vi "IEPE - Continuous  Input_tet.vi"() -> ()   [LabVIEW 2025]
doc: "This example demonstrates how to continuously acquire buffered acceleration, sound pressure, or force measurements from IEPE sensors using a DAQmx device.\n\nFor instructions on how to connect your signals to the DAQ device, refer to your device documentation."
uses:
  <vilib>/Math Plots/3D Math Plots/3D Contour/3D Contour XCtrl/3D Contour.xctl
  <vilib>/Utility/error.llb/DialogType.ctl
  <vilib>/DAQmx/read.llb/DAQmx Read (Analog 1D Wfm NChan NSamp).vi
  <vilib>/DAQmx/miscellaneous.llb/DAQmx Fill In Error Info.vi
  <vilib>/DAQmx/configure/trigger.llb/DAQmx Start Trigger (Digital Edge).vi
  <vilib>/DAQmx/configure/timing.llb/DAQmx Timing (Sample Clock).vi
  <vilib>/DAQmx/configure/task.llb/DAQmx Configure Logging (TDMS).vi
  <vilib>/DAQmx/create/channels.llb/DAQmx Create Channel (AI-Sound Pressure-Microphone).vi
  <vilib>/DAQmx/create/channels.llb/DAQmx Create Channel (AI-Force-IEPE Sensor).vi
  <vilib>/DAQmx/create/channels.llb/DAQmx Create Channel (AI-Acceleration-Accelerometer).vi
  <vilib>/DAQmx/configure/trigger.llb/DAQmx Start Trigger (Analog Edge).vi
  <vilib>/DAQmx/configure/trigger.llb/DAQmx Start Trigger (Time).vi
  <vilib>/Math Plots/3D Math Plots/3D Contour/3D Contour Datatype/Public/Plot Helper (Vector).vi
  <vilib>/Waveform/WDTOps.llb/WDT Waveform Duration DBL.vi
  <vilib>/Waveform/WDTOps.llb/WDT Append Waveforms DBL.vi
  <resource>/objmgr/daqmx.rc
  <vilib>/Math Plots/3D Math Plots/3D Contour/3D Contour Datatype/3D Contour Datatype.lvclass
panel:
  in  "last order plot":sgl
  in  "rotation speed":sgl
  out "3D-Kontur":refnum<class "3D Plot Datatype.lvclass">[](xcontrol)
  in  "filename":string
  in  "Dateipfad":path
  in  "on hold time (s)":u32=900
  out "FFT":cluster{dbl, "freq_step":dbl, "abs_FFT":dbl[]}(graph)
  in  "duration (s) control":dbl=30.0
  out "current duration":dbl caption="Dauer" format="%0.2f"
  in  "Trigger Type":T1(tab)
  in  "Digital Start Trigger Edge":i32(ring)=10280 caption="Edge" items=["Rising"=10280, "Falling"=10171]
  in  "Digital Start Trigger Source":tag="/Dev1/PFI0" caption="Source"
  in  "Digital Pause Trigger Pause When":i32(ring)=10192 caption="Pause When" items=["High"=10192, "Low"=10214]
  in  "Digital Pause Trigger Source":tag="/Dev1/PFI0" caption="Source"
  in  "Analog Start Trigger Level":dbl caption="Level" format="%0.2f"
  in  "Analog Start Trigger Hysteresis":dbl caption="Hysteresis" format="%.2f"
  in  "Analog Start Trigger Slope":i32(ring)=10280 caption="Slope" items=["Rising"=10280, "Falling"=10171]
  in  "Analog Start Trigger Source":string="APFI0" caption="Source"
  in  "Analog Pause Trigger Source":string="APFI0" caption="Source"
  in  "Analog Pause Trigger Pause When":i32(ring)=10093 caption="Pause When" items=["Above Level"=10093, "Below Level"=10107]
  in  "Analog Pause Trigger Level":dbl caption="Level" format="%.2f"
  in  "When":timestamp
  in  "Select Time\nManually":bool
  in  "IEPE Current Value (A)":dbl=0.004
  in  "IEPE Excitation Source":i32(ring)=10200 items=["Internal"=10200, "External"=10167, "None"=10230]
  in  "Terminal Configuration":i32(ring)=-1 items=["default"=-1, "RSE"=10083, "NRSE"=10078, "Differential"=10106, "Pseudodifferential"=12529]
  in  "Physical Channel":tag="cDAQ3Mod2/ai0"
  in  "Task Type":T2(tab)
  in  "Min Acceleration":dbl=-100.0
  in  "Max Acceleration":dbl=100.0
  in  "Sensitivity":dbl=50.0
  in  "Acceleration Units":i32(ring)=10186 items=["g"=10186, "m/s^2"=12470, "in/s^2"=12471, "From Custom Scale"=10065]
  in  "Sensitivity Units":i32(ring)=12509 items=["mVolts/g"=12509, "Volts/g"=12510]
  in  "Max Sound Pressure Level (dB)":dbl=120.0
  in  "Sound Pressure Units":i32(ring)=10081 items=["Pascals"=10081, "From Custom Scale"=10065]
  in  "Microphone Sensitivity":dbl=10.0
  in  "Sensitivity":dbl=50.0
  in  "Min Force":dbl=-100.0
  in  "Max Force":dbl=100.0
  in  "Sensitivity Units":i32(ring)=15891 items=["mVolts/N"=15891, "mVolts/lb"=15892]
  in  "Force Units":i32(ring)=15875 items=["Newtons"=15875, "Pounds"=15876, "From Custom Scale"=10065]
  in  "Stop":bool
  out "Waveform Graph":waveform(dbl)[](graph)
  in  "TDMS File Path":path
  in  "Samples per Loop":i32=100
  in  "Sample Rate":dbl=1000.0
  in  "Sample Clock Source":tag="OnboardClock"
  out "Actual Sample Rate":dbl=1000.0000111176631 format="%0.2f"
  in  "Logging Mode":i32(ring)=10231 items=["Off"=10231, "Log and Read"=15842]
  # "Channel Settings"
  # "Acquired Data"
  # "Trigger Settings"
  # "Timing Settings"
  # "Logging Settings"
  # "To enable triggers, select a tab above, and configure the settings.\n\nNot all hardware supports all trigger types. Refer to your device documentation for more information."
  # "This trigger type is not supported in continuous sample timing. \n\nRefer to your device documentation for more information on which triggers are supported."
  # "This trigger type is not supported in continuous sample timing. \n\nRefer to your device documentation for more information on which triggers are supported."
  # "If time is not manually set, task will begin after 10 seconds"
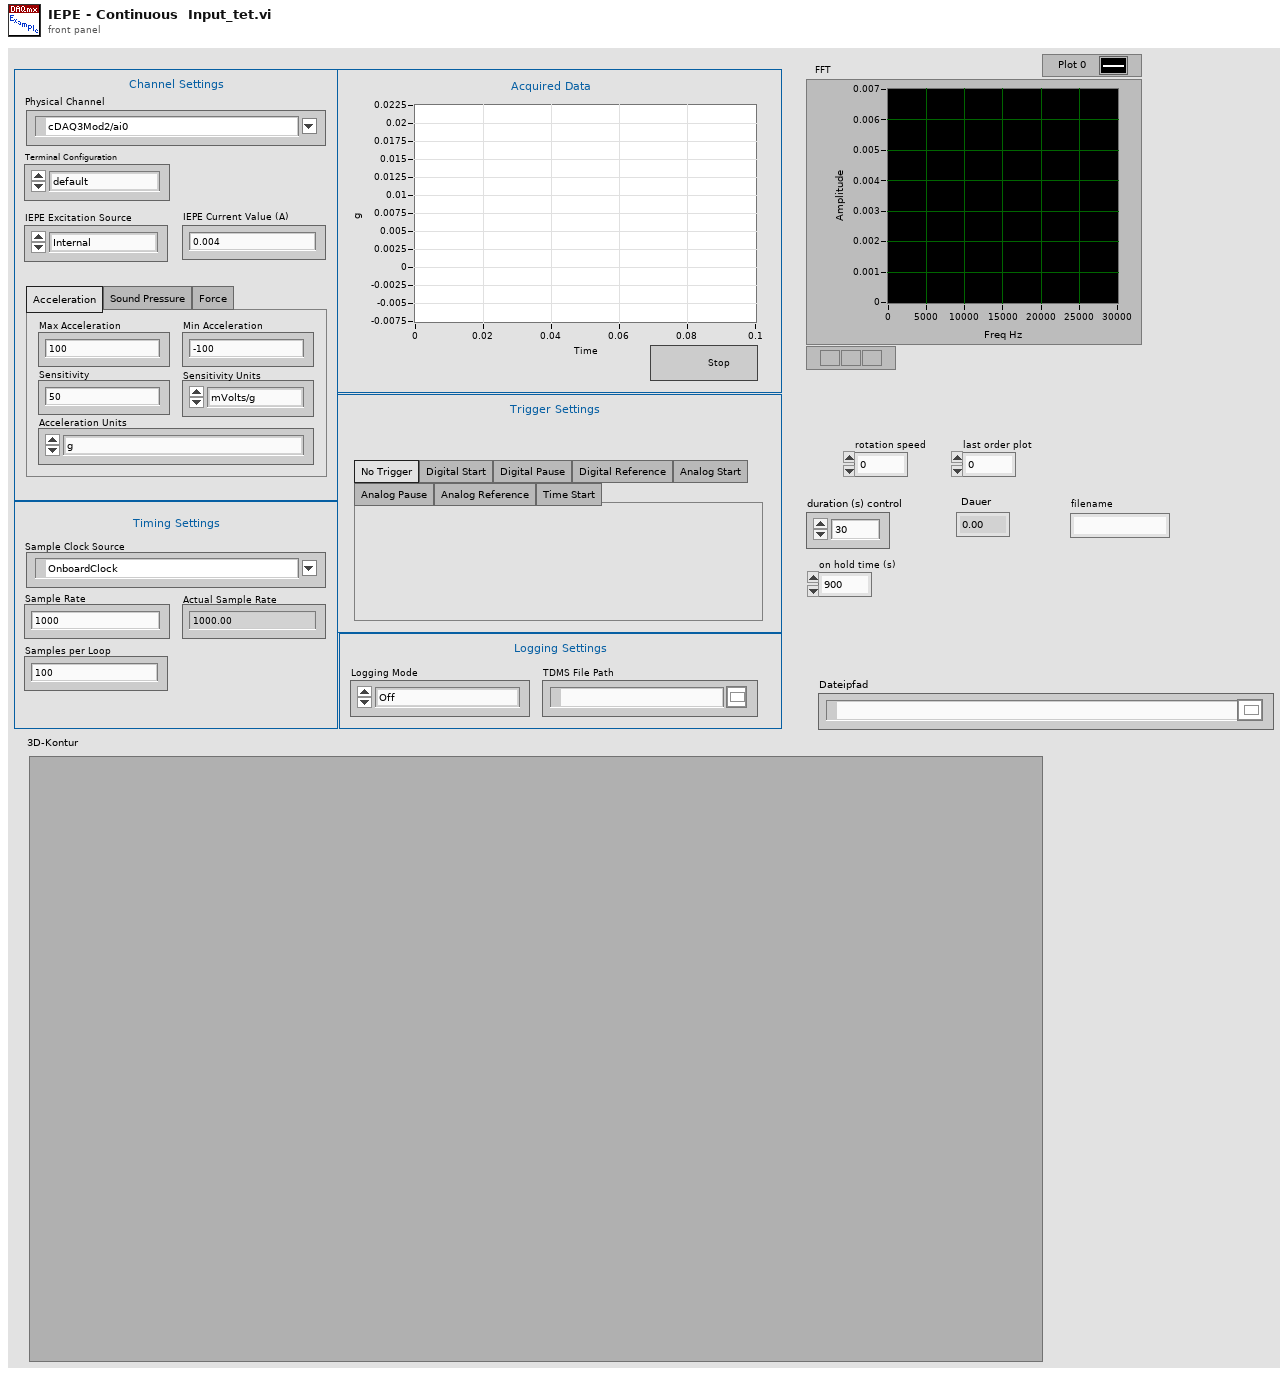
[diagram p1: front panel]
types:
  T1 = enum32{"No Trigger", "Digital Start", "Digital Pause", "Digital Reference", "Analog Start", "Analog Pause", "Analog Reference", "Time Start"}
  T2 = enum32{"Acceleration", "Sound Pressure", "Force"}
  T3 = typedef "DialogType.ctl" = u16
  T4 = cluster{"abs_FFT":dbl[], "frequencies":dbl[], "Huell_spec":dbl[], "Envelope":dbl[], "freq_step":dbl, "duration":dbl}
  T5 = enum16{"open", "open or create", "create or replace", "create", "open (read-only)"}
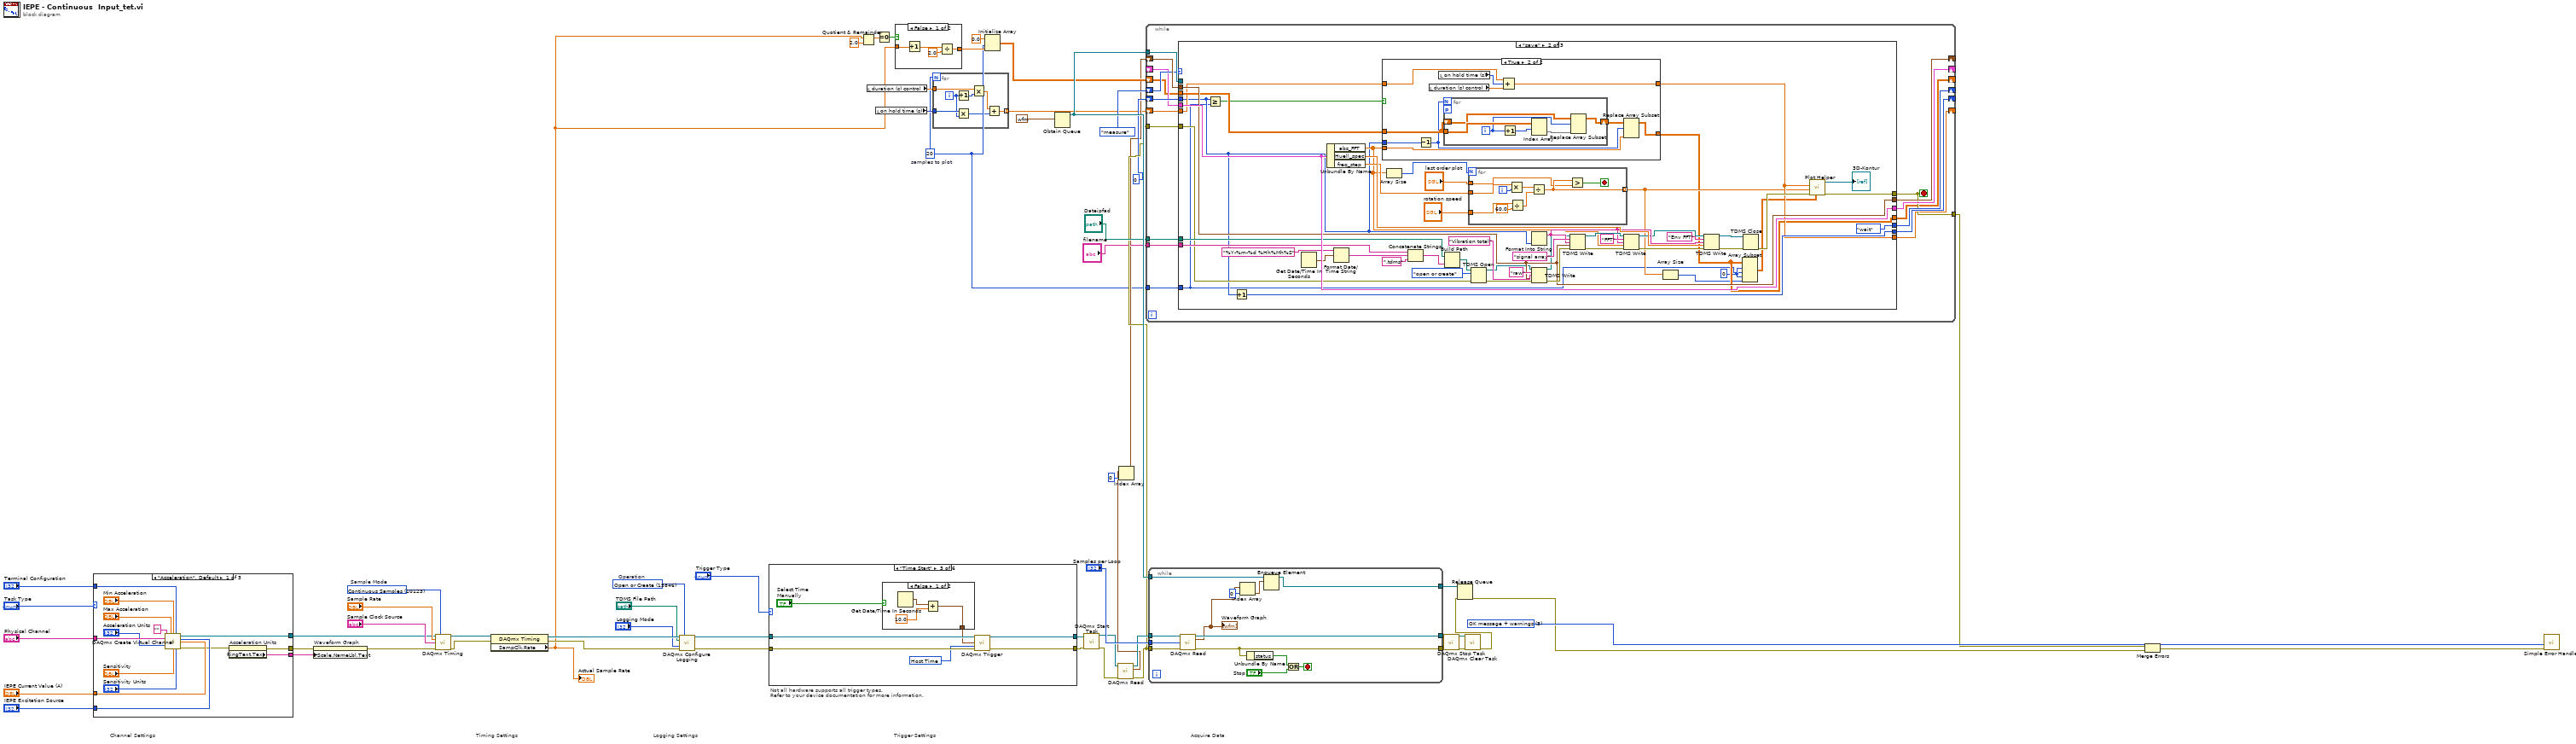
[diagram p0: block diagram]
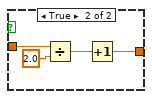
[diagram p2: hidden frame]
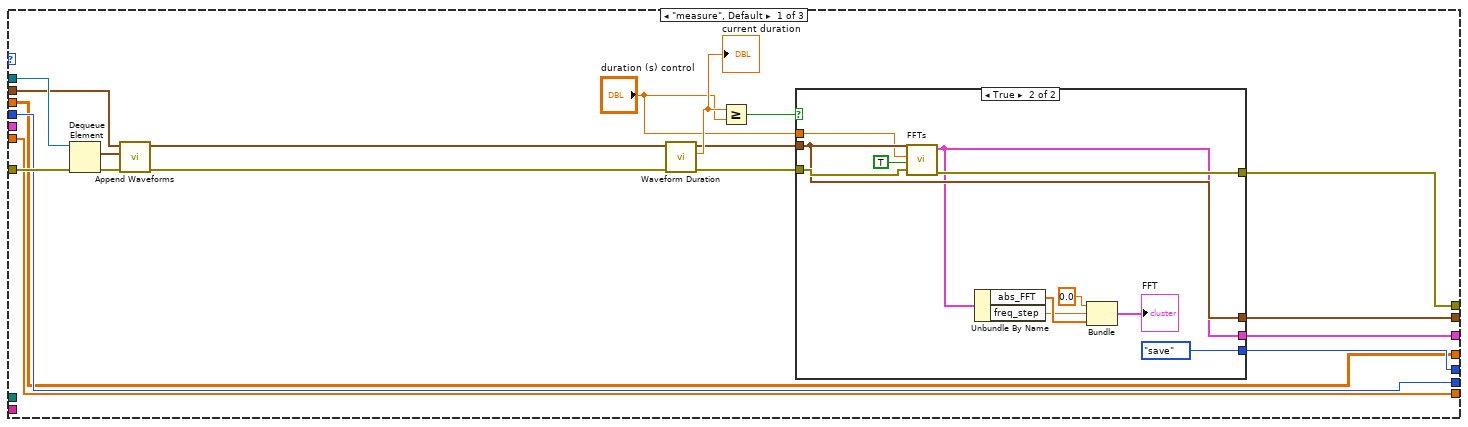
[diagram p3: hidden frame]
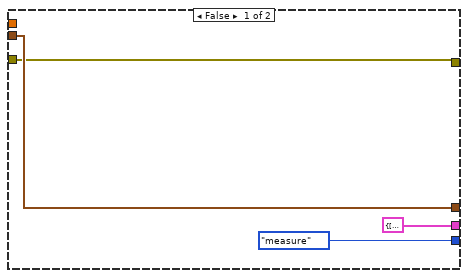
[diagram p4: hidden frame]
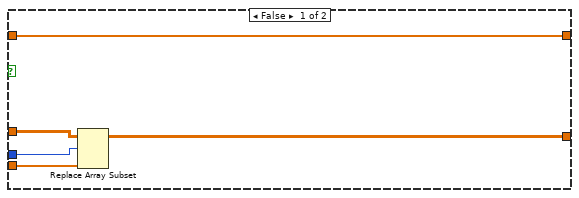
[diagram p5: hidden frame]
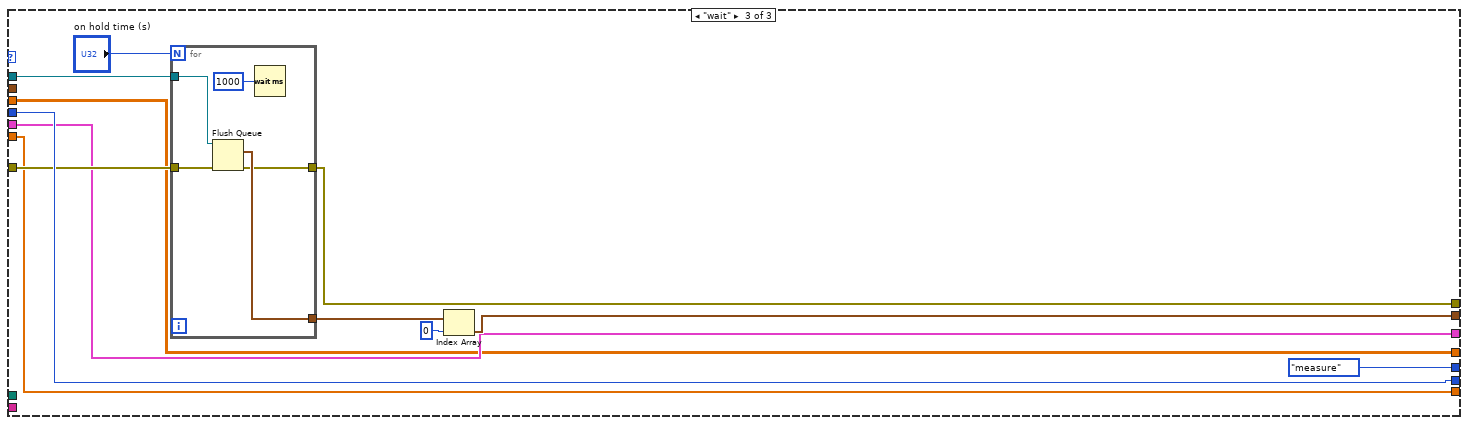
[diagram p6: hidden frame]
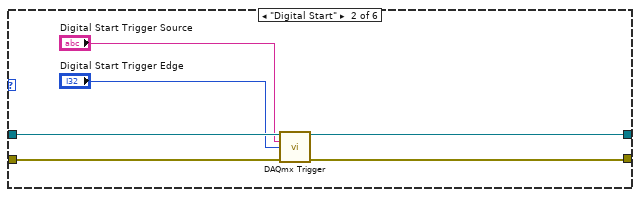
[diagram p8: hidden frame]
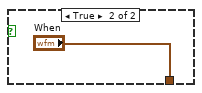
[diagram p9: hidden frame]
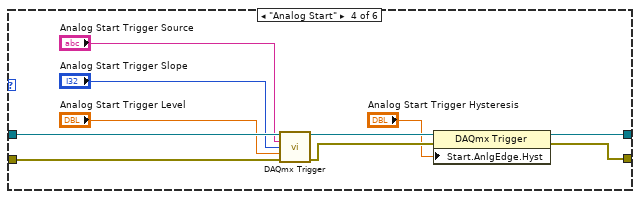
[diagram p10: hidden frame]
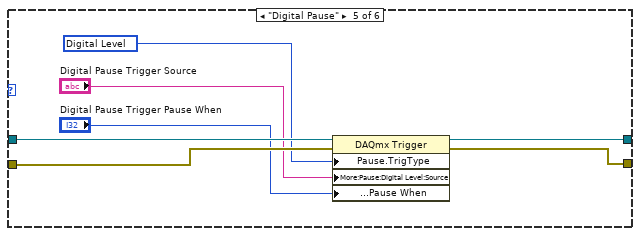
[diagram p11: hidden frame]
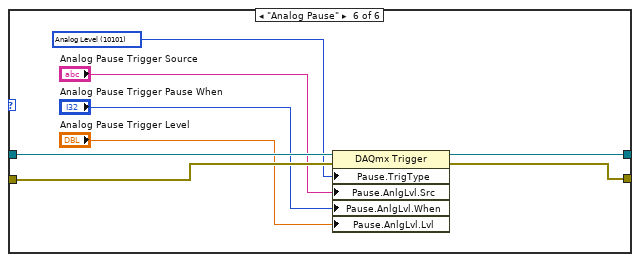
[diagram p12: hidden frame]
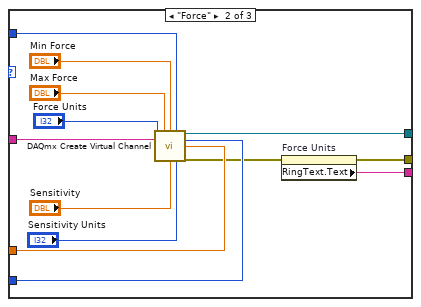
[diagram p13: hidden frame]
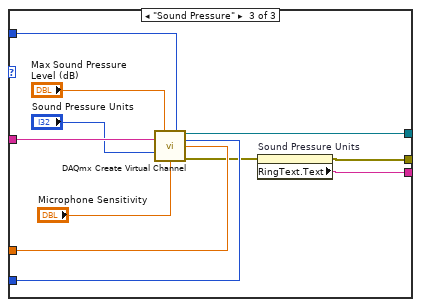
[diagram p14: hidden frame]
diagram:
  w1 = 20  # samples to plot
  w36 = T3 3 items=["no dialog", "OK message", "continue or stop message", "OK message + warnings", "continue/stop + warnings"] ("type of dialog (OK msg:1)")
  w54 = 15846 items=["Open"=10437, "Open or Create"=15846, "Create or Replace"=15847, "Create"=15848]  # Operation
  w57 = 10123 items=["Finite Samples"=10178, "Continuous Samples"=10123, "Hardware Timed Single Point"=12522]  # Sample Mode
  # "Trigger Settings"
  # "Not all hardware supports all trigger types.\nRefer to your device documentation for more information."
  # "Acquire Data"
  # "Timing Settings"
  # "Channel Settings"
  # "Logging Settings"
  n1 = case shown="\"Acceleration\", Default" "Task Type" {
    tunnel: [w63 w76 w90] -> w43
    tunnel: [w73 w86 w97] -> w44
    tunnel: "Physical Channel" -> [w72 w85 w96]
    tunnel: "IEPE Excitation Source" -> [w71 w84 w92]
    tunnel: "IEPE Current Value (A)" -> [w70 w83 w93]
    tunnel: "Terminal Configuration" -> [w69 w82 w95]
    tunnel: [w61 w75 w89] -> w42
    frame "Acceleration", Default {
      n2 = call-poly <vilib>:"DAQmx Create Virtual Channel.vi"("maximum value"="Max Acceleration", "minimum value"="Min Acceleration", "input terminal configuration"=w69, "physical channels"=w72, "current excitation source"=w71, "name to assign"="", "current excitation value"=w70, "units"="Acceleration Units", "sensitivity"="Sensitivity", "sensitivity units"="Sensitivity Units") -> ("task out"=w73:refnum<k21>, "error out"=w62:errorcluster)  [unwired: 4 in]
      n3 = property on="Acceleration Units" class="Ring (strict)"(error in=w62) -> (error out=w63:errorcluster, "RingText.Text"=w61:string)  [unwired: 1 in, 1 out]
    }
    frame "Force" {
      n4 = call-poly <vilib>:"DAQmx Create Virtual Channel.vi"("maximum value"="Max Force", "minimum value"="Min Force", "input terminal configuration"=w82, "physical channels"=w85, "current excitation source"=w84, "current excitation value"=w83, "units"="Force Units", "sensitivity"="Sensitivity", "sensitivity units"="Sensitivity Units") -> ("task out"=w86:refnum<k21>, "error out"=w74:errorcluster)  [unwired: 5 in]
      n5 = property on="Force Units" class="Ring (strict)"(error in=w74) -> (error out=w76:errorcluster, "RingText.Text"=w75:string)  [unwired: 1 in, 1 out]
    }
    frame "Sound Pressure" {
      n6 = call-poly <vilib>:"DAQmx Create Virtual Channel.vi"("maximum sound pressure level"="Max Sound Pressure Level (dB)", "input terminal configuration"=w95, "physical channels"=w96, "current excitation source"=w92, "current excitation value"=w93, "units"="Sound Pressure Units", "microphone sensitivity"="Microphone Sensitivity") -> ("task out"=w97:refnum<k21>, "error out"=w88:errorcluster)  [unwired: 7 in]
      n7 = property on="Sound Pressure Units" class="Ring (strict)"(error in=w88) -> (error out=w90:errorcluster, "RingText.Text"=w89:string)  [unwired: 1 in, 1 out]
    }
  }
  n8 = property on="Waveform Graph" class="WFGraph (strict)"(error in=w43, "YScale.NameLbl.Text"=w42) -> (error out=w41:errorcluster)  [unwired: 1 in, 1 out]
  n9 = call-poly <vilib>:"DAQmx Timing.vi"("task/channels in"=w44, "sample mode"=w57, "rate"="Sample Rate", "source"="Sample Clock Source", "error in"=w41) -> ("task out"=w59:refnum<k21>, "error out"=w58:errorcluster)  [unwired: 9 in]
  n10 = property class="DAQmx Timing"(reference=w59, error in=w58) -> (reference out=w56:refnum<k21>, error out=w55:errorcluster, "SampClk.Rate"=w14:dbl)
  "Actual Sample Rate" <- w14
  n11 = call-poly <vilib>:"DAQmx Configure Logging.vi"("task/channels in"=w56, "operation"=w54, "file path"="TDMS File Path", "logging mode"="Logging Mode", "error in"=w55) -> ("task out"=w33:refnum<k21>, "error out"=w34:errorcluster)  [unwired: 9 in]
  n12 = case shown="\"Time Start\"" "Trigger Type" {
    tunnel: w33 -> [w99 w105 w112 w126 w133 w141]
    tunnel: w34 -> [w98 w104 w111 w125 w130 w138]
    tunnel: [w99 w103 w110 w123 w132 w140] -> w31
    tunnel: [w98 w102 w109 w122 w131 w139] -> w32
    frame "No Trigger", Default {
    }
    frame "Digital Start" {
      n13 = call-poly <vilib>:"DAQmx Trigger.vi"("task/channels in"=w105, "source"="Digital Start Trigger Source", "edge"="Digital Start Trigger Edge", "error in"=w104) -> ("task out"=w103:refnum<k21>, "error out"=w102:errorcluster)  [unwired: 10 in]
    }
    frame "Time Start" {
      w106 = 16126 items=["Host Time"=16126, "I/O Device Time"=16127] ("timescale")
      n14 = case shown="False" "Select Time\nManually" {
        tunnel: [w114 "When"] -> w107
        frame False {
          n15 = Get Date/Time In Seconds() -> (seconds since 1Jan1904=w115:timestamp)
          n16 = Add(x=w115, y=10.0) -> (x+y=w114:timestamp)
        }
        frame True {
        }
      }
      n17 = call-poly <vilib>:"DAQmx Trigger.vi"("task/channels in"=w112, "when"=w107, "timescale"=w106, "error in"=w111) -> ("task out"=w110:refnum<k21>, "error out"=w109:errorcluster)  [unwired: 10 in]
    }
    frame "Analog Start" {
      n18 = call-poly <vilib>:"DAQmx Trigger.vi"("task/channels in"=w126, "source"="Analog Start Trigger Source", "slope"="Analog Start Trigger Slope", "level"="Analog Start Trigger Level", "error in"=w125) -> ("task out"=w121:refnum<k21>, "error out"=w120:errorcluster)  [unwired: 9 in]
      n19 = property class="DAQmx Trigger"(reference=w121, error in=w120, "Start.AnlgEdge.Hyst"="Analog Start Trigger Hysteresis") -> (reference out=w123:refnum<k21>, error out=w122:errorcluster)
    }
    frame "Digital Pause" {
      w129 = 10152 items=["Analog Level"=10101, "Analog Window"=10103, "Digital Level"=10152, "Digital Pattern"=10398, "None"=10230] ("Pause.TrigType")
      n20 = property class="DAQmx Trigger"(reference=w133, error in=w130, "Pause.TrigType"=w129, "More:Pause:Digital Level:Source"="Digital Pause Trigger Source", "More:Pause:Digital Level:Pause When"="Digital Pause Trigger Pause When") -> (reference out=w132:refnum<k21>, error out=w131:errorcluster)
    }
    frame "Analog Pause" {
      w137 = 10101 items=["Analog Level"=10101, "Analog Window"=10103, "Digital Level"=10152, "Digital Pattern"=10398, "None"=10230] ("Pause.TrigType")
      n21 = property class="DAQmx Trigger"(reference=w141, error in=w138, "Pause.TrigType"=w137, "Pause.AnlgLvl.Src"="Analog Pause Trigger Source", "Pause.AnlgLvl.When"="Analog Pause Trigger Pause When", "Pause.AnlgLvl.Lvl"="Analog Pause Trigger Level") -> (reference out=w140:refnum<k21>, error out=w139:errorcluster)
    }
  }
  n22 = Quotient & Remainder(x=w14, y=2.0) -> (x-y*floor(x/y)=w15:dbl)  [unwired: 1 out]
  n23 = local read "duration (s) control"() -> (w3:dbl)
  n24 = local read "on hold time (s)"() -> (w4:u32)
  n25 = Equal To 0?(x=w15) -> (x = 0?=w16:bool)
  n26 = case shown="False" w16 {
    tunnel: w14 -> [w144 w147]
    tunnel: [w142 w146] -> w13
    frame False {
      n27 = Increment(x=w144) -> (x+1=w143:dbl)
      n28 = Divide(x=w143, y=2.0) -> (x/y=w142:dbl)
    }
    frame True {
      n29 = Divide(x=w147, y=2.0) -> (x/y=w149:dbl)
      n30 = Increment(x=w149) -> (x+1=w146:dbl)
    }
  }
  n31 = for {
    N: w1 -> [_]
    tunnel: w4 -> [w156]
    tunnel: w3 -> [w153]
    tunnel: [w150] -> w2 mode=indexing
    i -> [w155]
    n32 = Increment(x=w155) -> (x+1=w154:i32)
    n33 = Multiply(x=w156, y=w155) -> (x*y=w151:u32)
    n34 = Multiply(x=w153, y=w154) -> (x*y=w152:dbl)
    n35 = Add(x=w152, y=w151) -> (x+y=w150:dbl)
  }
  n36 = Initialize Array(0.0 ("Element"), w1, w13) -> (w6:dbl[][])
  n37 = Obtain Queue(element data type=waveform(dbl) {"t0"=timestamp(0 s since 1904-01-01), "dt"=1.0, "Y"=[]} ("Element")) -> (queue out=w30:refnum<queue>)  [unwired: 4 in, 2 out]
  n38 = call <vilib>:"DAQmx Start Task.vi"("task/channels in"=w31, "error in"=w32) -> ("task out"=w26:refnum<k21>, "error out"=w25:errorcluster)  [unwired: 12 in]
  n39 = call-poly <vilib>:"DAQmx Read.vi"("task/channels in"=w26, "error in"=w25) -> ("task out"=w24:refnum<k21>, "data"=w21:waveform(dbl)[], "error out"=w18:errorcluster)  [unwired: 11 in]
  n40 = Index Array(array=w21, index=0) -> (element=w5:waveform(dbl))
  n41 = while {
    tunnel: w30 -> [w174]
    tunnel: w18 -> [w173]
    shift-right: [w172] -> _
    shift-left: w5 -> [w171]
    shift-right: [w170] -> _
    shift-left: _ -> [w165]
    shift-right: [w168] -> _
    shift-left: enum16{"measure", "save", "wait"}."measure" -> [w169]
    shift-right: [w166] -> _
    shift-left: 0 -> [w167]
    tunnel: [w164] -> w11
    tunnel: "Dateipfad" -> [w163]
    tunnel: "filename" -> [w162]
    shift-right: [w160] -> _
    shift-left: w6 -> [w161]
    tunnel: w1 -> [w158]
    shift-right: [w157] -> _
    shift-left: w2 -> [w159]
    stop <- w164 stop-if-true
    n42 = case shown="\"save\"" w169 {
      tunnel: w174 -> [w193 _ w298]
      tunnel: w173 -> [w192 w231 w299]
      tunnel: [w189 w244 w296] -> w172
      tunnel: [w188 w226 w292] -> w164
      tunnel: w171 -> [w186 w244 _]
      tunnel: [w182 w245 w293] -> w170
      tunnel: [w181 enum16{"measure", "save", "wait"}."wait" enum16{"measure", "save", "wait"}."measure"] -> w168
      tunnel: w167 -> [w180 w216 w300]
      tunnel: [w180 w254 w300] -> w166
      tunnel: w165 -> [_ w245 w293]
      tunnel: w163 -> [_ w233 _]
      tunnel: w162 -> [_ w239 _]
      tunnel: w161 -> [w179 w222 w290]
      tunnel: [w179 w213 w290] -> w160
      tunnel: w159 -> [w175 w218 w289]
      tunnel: w158 -> [_ w209 _]
      tunnel: [w175 w217 w289] -> w157
      frame "measure", Default {
        n43 = Dequeue Element(queue=w193, error in (no error)=w192) -> (element=w187:waveform(dbl), error out=w178:errorcluster)  [unwired: 1 in, 2 out]
        n44 = call-poly <vilib>:"Append Waveforms.vi"("error in (no error)"=w178, "waveform B"=w187, "waveform A"=w186) -> ("error out"=w177:errorcluster, "waveform out"=w185:waveform(dbl))  [unwired: 7 in]
        n45 = call-poly <vilib>:"Waveform Duration.vi"("error in (no error)"=w177, "waveform in"=w185) -> ("error out"=w176:errorcluster, "duration"=w191:dbl, "waveform out"=w184:waveform(dbl))  [unwired: 7 in]
        "current duration" <- w191
        n46 = Greater Or Equal?(x=w191, y="duration (s) control") -> (x >= y?=w190:bool)
        n47 = case shown="True" w190 {
          tunnel: w176 -> [w196 w206]
          tunnel: w184 -> [w197 w203]
          tunnel: [w197 w203] -> w189
          tunnel: [w196 w204] -> w188
          tunnel: "duration (s) control" -> [_ w202]
          tunnel: [T4 {"abs_FFT"=[], "frequencies"=[], "Huell_spec"=[], "Envelope"=[], "freq_step"=0.0, "duration"=0.0} ("output cluster") w199] -> w182
          tunnel: [enum16{"measure", "save", "wait"}."measure" enum16{"measure", "save", "wait"}."save"] -> w181
          frame False {
          }
          frame True {
            n48 = call "FFTs.vi"("error in"=w206, "Envelope&Hu?"=TRUE, "duration"=w202, "waveform in"=w203) -> ("error out"=w204:errorcluster, "output cluster"=w199:T4)  [unwired: 6 in]
            n49 = Unbundle By Name(w199) -> ("abs_FFT"=w208:dbl[], "freq_step"=w205:dbl)
            n50 = Bundle(0.0, "freq_step"=w205, "abs_FFT"=w208) -> (→"FFT":cluster{dbl, "freq_step":dbl, "abs_FFT":dbl[]})  [unwired: 1 in]
          }
        }
      }
      frame "save" {
        w212 = 0 ("length")
        n51 = Greater Or Equal?(x=w216, y=w209) -> (x >= y?=w220:bool)
        n52 = Increment(x=w216) -> (x+1=w254:i32)
        n53 = Get Date/Time In Seconds() -> (seconds since 1Jan1904=w238:timestamp)
        n54 = Unbundle By Name(w245) -> ("abs_FFT"=w221:dbl[], "Huell_spec"=w250:dbl[], "freq_step"=w223:dbl)
        n55 = Format Date/Time String(time format string (%c)="%Y-%m-%d %Hh%Mh%S" ("Zeitformatierungs-String (%c)"), seconds (now)=w238) -> (date/time string=w236:string)  [unwired: 1 in]
        n56 = case shown="True" w220 {
          tunnel: w216 -> [w260 w273]
          tunnel: w222 -> [w263 w272]
          tunnel: w221 -> [w261 w269]
          tunnel: [w262 w268] -> w213
          tunnel: w218 -> [w259 w267]
          tunnel: [w259 w266] -> w217
          frame False {
            n57 = Replace Array Subset(array=w263, new element=w261, index (row)=w260) -> (w262:dbl[][])  [unwired: 1 in]
          }
          frame True {
            n58 = Decrement(x=w273) -> (x-1=w270:i32)
            n59 = local read "duration (s) control"() -> (w264:dbl)
            n60 = local read "on hold time (s)"() -> (w265:u32)
            n61 = for {
              N: w270 -> [_]
              tunnel: w272 -> [w279]
              shift-right: [w274] -> w271
              shift-left: w272 -> [w276]
              workers-P: _ -> [_]
              i -> [w275]
              n62 = Increment(x=w275) -> (x+1=w278:i32)
              n63 = Index Array(array=w279, index (row)=w278) -> (element=w277:dbl[])  [unwired: 1 in]
              n64 = Replace Array Subset(array=w276, new element=w277, index (row)=w275) -> (w274:dbl[][])  [unwired: 1 in]
            }
            n65 = Compound Arithmetic op=ADD(w267, w265, w264) -> (w266:dbl[])
            n66 = Replace Array Subset(array=w271, new element=w269, index (row)=w270) -> (w268:dbl[][])  [unwired: 1 in]
          }
        }
        n67 = Array Size(array=w221) -> (size(s)=w224:i32)
        n68 = Concatenate Strings(w239, w236, ".tdms" ("String")) -> (w234:string)
        n69 = Build Path(base path=w233, name or relative path=w234) -> (appended path=w232:path)
        n70 = for {
          N: w224 -> [_]
          tunnel: w223 -> [w287]
          tunnel: [w282] -> w214 mode=indexing
          tunnel: "rotation speed" -> [w283]
          tunnel: "last order plot" -> [w281]
          i -> [w288]
          stop <- w280 stop-if-true
          n71 = Multiply(x=w287, y=w288) -> (x*y=w284:dbl)
          n72 = Divide(x=w283, y=sgl 60.0) -> (x/y=w285:sgl)
          n73 = Divide(x=w284, y=w285) -> (x/y=w282:dbl)
          n74 = Greater?(x=w282, y=w281) -> (0:w280:bool)
        }
        n75 = TDMS Open(8:w231, 10:T5."open or create" ("Operation (0:open)"), 11:w232) -> (0:w230:errorcluster, 3:w240:refnum<k34>)  [unwired: 4 in]
        n76 = Format Into String(w216) -> (resulting string=w248:string)  [unwired: 3 in, 1 out]
        n77 = TDMS Write(0:w240, 5:"raw" ("Gruppenname (Eingang, Unbenannt)"), 7:"Vibration total" ("Kanalnamen (Eingang, unbenannt)"), 9:w244, 11:w230) -> (4:w243:refnum<k34>, 15:w253:errorcluster)  [unwired: 1 in, 2 out]
        n78 = TDMS Write(0:w243, 5:"signal array" ("Gruppenname (Eingang, Unbenannt)"), 7:w248, 9:w244, 11:w253) -> (4:w252:refnum<k34>, 15:w247:errorcluster)  [unwired: 1 in, 2 out]
        n79 = TDMS Write(0:w252, 5:"FFT" ("Gruppenname (Eingang, Unbenannt)"), 7:w248, 9:w221, 11:w247) -> (4:w242:refnum<k34>, 15:w246:errorcluster)  [unwired: 1 in, 2 out]
        n80 = Array Size(array=w214) -> (size(s)=w211:i32)
        n81 = TDMS Write(0:w242, 5:"Env FFT" ("Gruppenname (Eingang, Unbenannt)"), 7:w248, 9:w250, 11:w246) -> (4:w229:refnum<k34>, 15:w228:errorcluster)  [unwired: 1 in, 2 out]
        n82 = Array Subset(array=w213, index (row)=w212, length (row)=w209, index (col)=w212, length (col)=w211) -> (w210:dbl[][])
        n83 = TDMS Close(8:w228, 11:w229) -> (0:w227:errorcluster)  [unwired: 1 out]
        n84 = call-poly <vilib>:"Plot Helper.vi"("z matrix"=w210, "error in (no error)"=w227, "y vector"=w214, "x vector"=w217) -> ("error out"=w226:errorcluster, "3D Plot lvclass Array out"=→"3D-Kontur":refnum<class "3D Plot Datatype.lvclass">[])  [unwired: 2 in, 4 out]
      }
      frame "wait" {
        n85 = for {
          N: "on hold time (s)" -> [_]
          tunnel: w299 -> [w304]
          tunnel: w298 -> [w303]
          tunnel: [w302] -> w297
          tunnel: [w301] -> w292
          n86 = Flush Queue(queue=w303, error in (no error)=w304) -> (remaining elements=w302:waveform(dbl)[], error out=w301:errorcluster)  [unwired: 1 out]
          n87 = Wait (ms)(milliseconds to wait=u32 1000 ("Zu wartende ms")) -> ()  [unwired: 1 out]
        }
        n88 = Index Array(array=w297, index=0 ("Index")) -> (element=w296:waveform(dbl))
      }
    }
  }
  n89 = while {
    tunnel: w24 -> [w318]
    tunnel: w18 -> [w317]
    tunnel: [w310] -> w37
    tunnel: [w315] -> w38
    tunnel: w30 -> [w308]
    tunnel: [w307] -> w29
    tunnel: "Samples per Loop" -> [w306]
    stop <- w316 stop-if-true
    n90 = call-poly <vilib>:"DAQmx Read.vi"("task/channels in"=w318, "number of samples per channel"=w306, "error in"=w317) -> ("task out"=w315:refnum<k21>, "data"=w312:waveform(dbl)[], "error out"=w310:errorcluster)  [unwired: 10 in]
    "Waveform Graph" <- w312
    n91 = Index Array(array=w312, index=0) -> (element=w309:waveform(dbl))
    n92 = Unbundle By Name(w310) -> ("status"=w314:bool)
    n93 = Enqueue Element(queue=w308, element=w309) -> (queue out=w307:refnum<queue>)  [unwired: 2 in, 2 out]
    n94 = Or(x=w314, y="Stop") -> (x .or. y?=w316:bool)
  }
  n95 = call <vilib>:"DAQmx Stop Task.vi"("task/channels in"=w38, "error in"=w37) -> ("task out"=w40:refnum<k21>, "error out"=w39:errorcluster)  [unwired: 12 in]
  n96 = call <vilib>:"DAQmx Clear Task.vi"("task in"=w40, "error in"=w39) -> ("error out"=w28:errorcluster)  [unwired: 13 in]
  n97 = Release Queue(queue=w29, error in (no error)=w28) -> (error out=w10:errorcluster)  [unwired: 1 in, 2 out]
  n98 = Merge Errors(w11, w10) -> (w9:errorcluster)
  n99 = call <vilib>:"Simple Error Handler.vi"("type of dialog (OK msg:1)"=w36, "error in (no error)"=w9) -> ()  [unwired: 3 in, 5 out]
